vi "Measure X Delta.vi"(8 "error in":errorcluster) -> (0 "error out":errorcluster, 2 "X Delta":dbl format="%_6e")   [LabVIEW 2009]
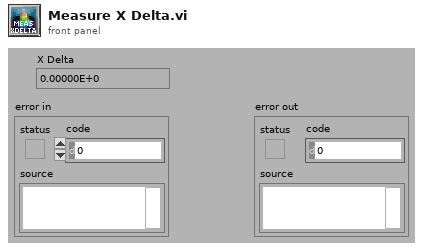
[diagram p1: front panel]
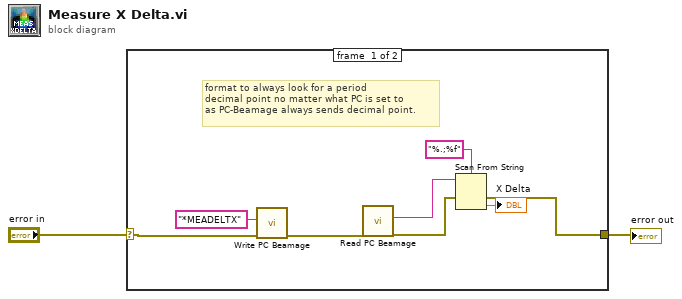
[diagram p0: block diagram]
diagram:
  n1 = case shown="No Error" "error in" {
    selector: "error in" -> [w7 w11]
    tunnel: [w4 w11] -> w1
    frame #0 {
      # "format to always look for a period\ndecimal point no matter what PC is set to\nas PC-Beamage always sends decimal point."
      n2 = call "Write PC Beamage.vi"("error in"=w7, "command"="*MEADELTX") -> ("error out"=w6:errorcluster)  [unwired: 9 in]
      n3 = call "Read PC Beamage.vi"("error in"=w6) -> ("error out"=w5:errorcluster, "Reply"=w10:string)  [unwired: 9 in]
      n4 = Scan From String(format string="%.;%f", input string=w10, error in=w5) -> (error out=w4:errorcluster, output 1=→"X Delta":dbl)  [unwired: 2 in, 2 out]
    }
    frame #1 {
    }
  }
  "error out" <- w1
